vi "seti_labview_read_power_spectrum.vi"(8 "error in (no error)":errorcluster, 11 "Power Spectrum Data file path":path) -> (0 "error out":errorcluster, 3 "Array of Power Spectrum Data":T1[](array[typedef]))   [LabVIEW 2014, in "SETI_LV.lvlib"]
uses:
  SETI_LV/SETI_LV.lvlib
  Power Spectrum Data.ctl
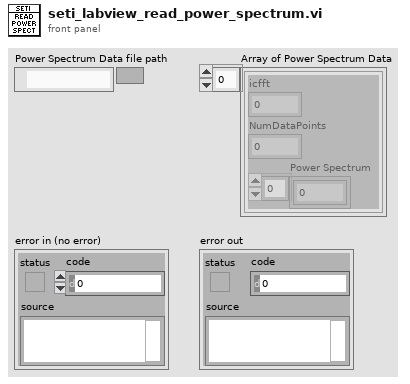
[diagram p1: front panel]
types:
  T1 = typedef "SETI_LV.lvlib/Power Spectrum Data.ctl" = cluster{"icfft":i32, "NumDataPoints":i32, "Power Spectrum":sgl[]}
  T2 = enum16{"big-endian, network order", "native, host order", "little-endian"}
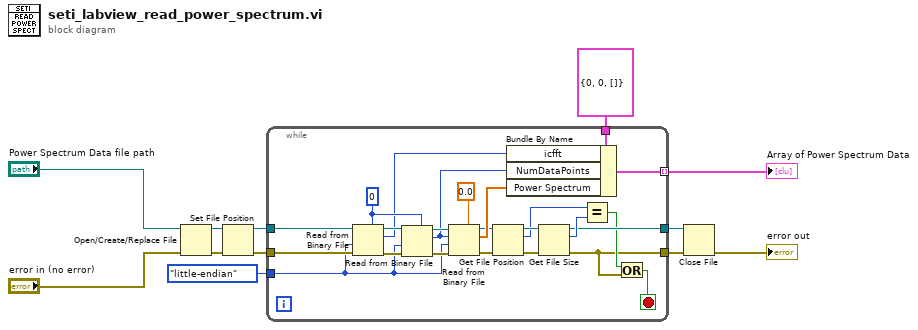
[diagram p0: block diagram]
diagram:
  n1 = Open/Create/Replace File(file path (use dialog)="Power Spectrum Data file path", error in="error in (no error)") -> (refnum out=w2:refnum<file>, error out=w5:errorcluster)  [unwired: 4 in, 1 out]
  n2 = Set File Position(refnum=w2, error in=w5) -> (refnum out=w4:refnum<file>, error out=w6:errorcluster)  [unwired: 2 in]
  n3 = while {
    tunnel: T2."little-endian" ("byte order (0:big-endian, network order)") -> [w28]
    tunnel: w6 -> [w35]
    tunnel: w4 -> [w34]
    tunnel: T1 {"icfft"=0, "NumDataPoints"=0, "Power Spectrum"=[]} -> [w27]
    tunnel: [w23] -> w11 mode=indexing
    tunnel: [w13] -> w9
    tunnel: [w16] -> w10
    stop <- w14 stop-if-true
    w33 = 0
    n4 = Read from Binary File(5:w33, 8:w35, 9:w28, 11:w34) -> (0:w30:errorcluster, 2:w26:i32, 3:w29:refnum<file>)  [unwired: 2 in, 1 out]
    n5 = Read from Binary File(5:w33, 8:w30, 9:w28, 11:w29) -> (0:w31:errorcluster, 2:w25:i32, 3:w32:refnum<file>)  [unwired: 2 in, 1 out]
    n6 = Read from Binary File(5:sgl 0.0, 8:w31, 9:w28, 10:w25, 11:w32) -> (0:w17:errorcluster, 2:w24:sgl[], 3:w18:refnum<file>)  [unwired: 1 in, 1 out]
    n7 = Get File Position(4:w17, 7:w18) -> (0:w22:errorcluster, 2:w20:i64, 3:w21:refnum<file>)
    n8 = Bundle By Name(cluster=w27, "icfft"=w26, "NumDataPoints"=w25, "Power Spectrum"=w24) -> (w23:T1)
    n9 = Get File Size(file=w21, error in=w22) -> (refnum out=w16:refnum<file>, size (in bytes)=w19:i64, 0:w13:errorcluster)
    n10 = Equal?(x=w20, y=w19) -> (x = y?=w15:bool)
    n11 = Or(x=w15, y=w13) -> (x .or. y?=w14:bool)
  }
  "Array of Power Spectrum Data" <- w11
  n12 = Close File(refnum=w10, error in=w9) -> (error out=→"error out":errorcluster)  [unwired: 1 out]
